vi "IPS120 WH1 - Sweep Status.vi"(0 "Sweep Status":enum16{"Hold", "To Setpoint", "To Zero"}(ring)=enum."To Zero", 1 "GPIB Address":string) -> ()   [LabVIEW 2010]
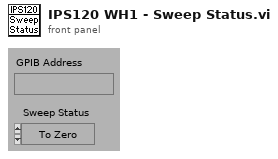
[diagram p1: front panel]
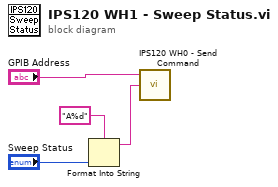
[diagram p0: block diagram]
diagram:
  n1 = Format Into String(format string="A%d", "Sweep Status") -> (resulting string=w1:string)  [unwired: 2 in, 1 out]
  n2 = call "IPS120 WH0 - Send Command.vi"("Command String"=w1, "VISA Address"="GPIB Address") -> ()  [unwired: 1 in, 3 out]
